vi "writeConfig.vi"   [LabVIEW 2018]
uses:
  <vilib>/Utility/error.llb/DialogType.ctl
  <vilib>/Utility/config.llb/Write Key (U32).vi
  <vilib>/Utility/config.llb/Write Key (Boolean).vi
  <vilib>/Utility/config.llb/Write Key (String).vi
  <vilib>/Utility/config.llb/NI_LVConfig.lvlib
types:
  T1 = typedef "DialogType.ctl" = u16
  T2 = typedef "NI_LVConfig.lvlib/Config Data RefNum.ctl" = refnum<k1>
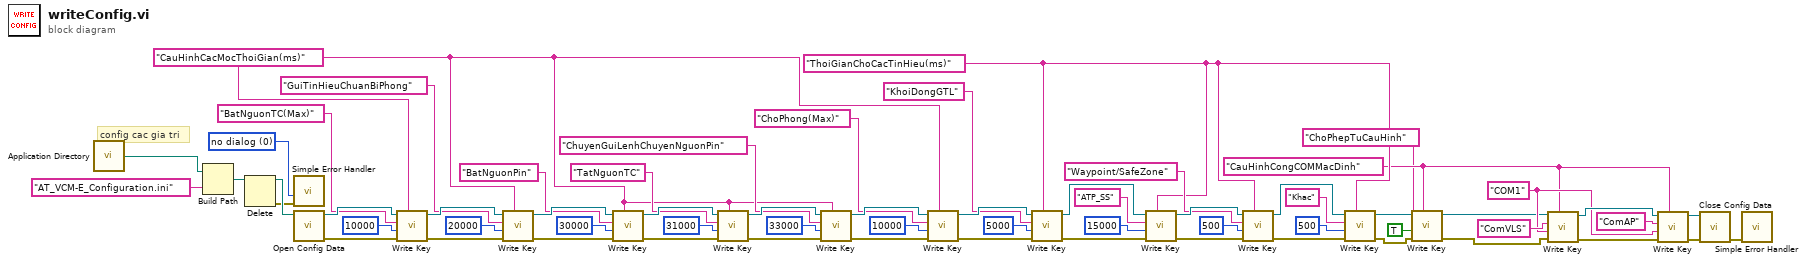
[diagram p0: block diagram]
diagram:
  w8 = "COM1" ("key")
  w7 = "CauHinhCongCOMMacDinh" ("key")
  w16 = T1 0 items=["no dialog", "OK message", "continue or stop message", "OK message + warnings", "continue/stop + warnings"] ("type of dialog (OK msg:1)")
  w29 = "ThoiGianChoCacTinHieu(ms)" ("key")
  w37 = "CauHinhCacMocThoiGian(ms)" ("key")
  # "config cac gia tri"
  n1 = call <vilib>:"Application Directory.vi"() -> ("Application Directory"=w15:path)
  n2 = Build Path(base path=w15, name or relative path="AT_VCM-E_Configuration.ini") -> (appended path=w62:path)
  n3 = Delete(path (use dialog)=w62) -> (deleted path=w61:path, error out=w17:errorcluster)  [unwired: 4 in, 1 out]
  n4 = call <vilib>:"Simple Error Handler.vi"("type of dialog (OK msg:1)"=w16, "error in (no error)"=w17) -> ()  [unwired: 1 in, 7 out]
  n5 = call <vilib>:"Open Config Data.vi"("configuration file path"=w61) -> ("error out"=w59:errorcluster, "refnum"=w60:T2)  [unwired: 2 in, 7 out]
  n6 = call-poly <vilib>:"Write Key.vi"("section"=w37, "error in (no error)"=w59, "value"=u32 10000, "key"="BatNguonTC(Max)", "refnum"=w60) -> ("error out"=w56:errorcluster, "refnum out"=w55:T2)  [unwired: 4 in, 1 out]
  n7 = call-poly <vilib>:"Write Key.vi"("section"=w37, "error in (no error)"=w56, "value"=u32 20000, "key"="GuiTinHieuChuanBiPhong", "refnum"=w55) -> ("error out"=w19:errorcluster, "refnum out"=w52:T2)  [unwired: 4 in, 1 out]
  n8 = call-poly <vilib>:"Write Key.vi"("section"=w37, "error in (no error)"=w19, "value"=u32 30000, "key"="BatNguonPin", "refnum"=w52) -> ("error out"=w20:errorcluster, "refnum out"=w49:T2)  [unwired: 4 in, 1 out]
  n9 = call-poly <vilib>:"Write Key.vi"("section"=w37, "error in (no error)"=w20, "value"=u32 31000, "key"="TatNguonTC", "refnum"=w49) -> ("error out"=w21:errorcluster, "refnum out"=w46:T2)  [unwired: 4 in, 1 out]
  n10 = call-poly <vilib>:"Write Key.vi"("section"=w37, "error in (no error)"=w21, "value"=u32 33000, "key"="ChuyenGuiLenhChuyenNguonPin", "refnum"=w46) -> ("error out"=w22:errorcluster, "refnum out"=w43:T2)  [unwired: 4 in, 1 out]
  n11 = call-poly <vilib>:"Write Key.vi"("section"=w37, "error in (no error)"=w22, "value"=u32 10000, "key"="ChoPhong(Max)", "refnum"=w43) -> ("error out"=w23:errorcluster, "refnum out"=w40:T2)  [unwired: 4 in, 1 out]
  n12 = call-poly <vilib>:"Write Key.vi"("section"=w29, "error in (no error)"=w23, "value"=u32 5000, "key"="KhoiDongGTL", "refnum"=w40) -> ("error out"=w24:errorcluster, "refnum out"=w36:T2)  [unwired: 4 in, 1 out]
  n13 = call-poly <vilib>:"Write Key.vi"("section"=w29, "error in (no error)"=w24, "value"=u32 15000, "key"="ATP_SS", "refnum"=w36) -> ("error out"=w25:errorcluster, "refnum out"=w33:T2)  [unwired: 4 in, 1 out]
  n14 = call-poly <vilib>:"Write Key.vi"("section"=w29, "error in (no error)"=w25, "value"=u32 500, "key"="Waypoint/SafeZone", "refnum"=w33) -> ("error out"=w26:errorcluster, "refnum out"=w30:T2)  [unwired: 4 in, 1 out]
  n15 = call-poly <vilib>:"Write Key.vi"("section"=w29, "error in (no error)"=w26, "value"=u32 500, "key"="Khac", "refnum"=w30) -> ("error out"=w1:errorcluster, "refnum out"=w4:T2)  [unwired: 4 in, 1 out]
  n16 = call-poly <vilib>:"Write Key.vi"("section"=w7, "error in (no error)"=w1, "value"=TRUE, "key"="ChoPhepTuCauHinh", "refnum"=w4) -> ("error out"=w2:errorcluster, "refnum out"=w3:T2)  [unwired: 4 in, 1 out]
  n17 = call-poly <vilib>:"Write Key.vi"("section"=w7, "error in (no error)"=w2, "value"=w8, "key"="ComVLS", "refnum"=w3) -> ("error out"=w11:errorcluster, "refnum out"=w13:T2)  [unwired: 4 in, 1 out]
  n18 = call-poly <vilib>:"Write Key.vi"("section"=w7, "error in (no error)"=w11, "value"=w8, "key"="ComAP", "refnum"=w13) -> ("error out"=w10:errorcluster, "refnum out"=w12:T2)  [unwired: 4 in, 1 out]
  n19 = call <vilib>:"Close Config Data.vi"("error in (no error)"=w10, "refnum"=w12) -> ("error out"=w27:errorcluster)  [unwired: 1 in, 8 out]
  n20 = call <vilib>:"Simple Error Handler.vi"("error in (no error)"=w27) -> ()  [unwired: 2 in, 7 out]
